vi "Request Data Persistence.vi"(6 "One Shot? (F)":bool, 7 "Initialize Persistence If None Found? (T)":bool=TRUE, 8 "error in (no error)":errorcluster, 9 "Data Type/Initial Value":variant, 10 "Datum Name":string, 11 "IObserver in":refnum<class "IObserver.lvclass">) -> (0 "error out":errorcluster, 2 "Subscription Policy":T1, 3 "IObserver out":refnum<class "IObserver.lvclass">)   [LabVIEW 2015, in "IObserver.lvlib" / "IObserver.lvclass"]
doc: "<License>\nCopyright © 2017 Composed Systems, LLC | All rights reserved\nwww.composed.io\n\nAuthor: Ethan Stern <ethan.stern@composed.io>\n\nThis software is provided \"AS IS\" WITHOUT WARRANTIES, either express or implied, AND IS FOR EDUCATIONAL PURPOSES ONLY.\n</License>"
uses:
  IObserver.lvclass
  IMediator/ISubscriptionPolicy/ISubscriptionPolicy Reference.ctl
  IMediator/ISubscriptionPolicy/ISubscriptionPolicy.lvclass
  <vilib>/ActorFramework/Actor/Actor.lvclass/Actor.ctl
  <vilib>/ActorFramework/Message Enqueuer/Message Enqueuer.lvclass/Message Enqueuer.ctl
  SubscriptionPolicy/ValueChangeSubscription/ValueChangeSubscription.lvclass/ValueChangeSubscription.ctl
  SubscriptionPolicy/OneShotSubscription/OneShotSubscription.lvclass/OneShotSubscription.ctl
  Transport/PersistToDiskTransport/PersistToDiskTransport.lvclass/PersistToDiskTransport.ctl
  IMediator/SubscriptionRequest/SubscriptionRequest.lvclass/SubscriptionRequest.ctl
  IObserver Messages/Subscribe Msg/Subscribe Msg.lvclass/Subscribe Msg.ctl
  <vilib>/ActorFramework/Message Enqueuer/Init from Existing Queue.vi
  <vilib>/ActorFramework/Message Enqueuer/Enqueue.vi
  <vilib>/Utility/error.llb/Clear Errors.vi
  <vilib>/ActorFramework/Message Priority Queue/Priority Enqueue.vi
  IObserver Messages/Subscribe Msg/Subscribe Msg.lvclass
  <vilib>/ActorFramework/Message Enqueuer/Message Enqueuer.lvclass
  IMediator/SubscriptionRequest/SubscriptionRequest.lvclass
  Transport/PersistToDiskTransport/PersistToDiskTransport.lvclass
  SubscriptionPolicy/OneShotSubscription/OneShotSubscription.lvclass
  SubscriptionPolicy/ValueChangeSubscription/ValueChangeSubscription.lvclass
  <vilib>/ActorFramework/Actor/Actor.lvclass
panel:
  in  "Persistence Folder Path":path
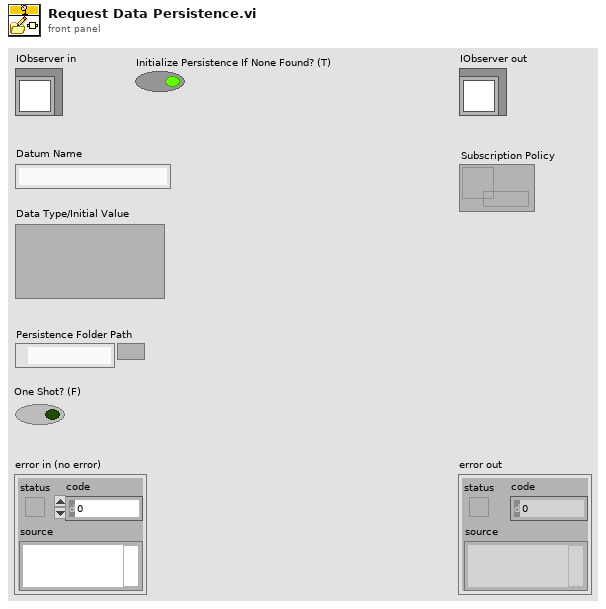
[diagram p1: front panel]
types:
  T1 = typedef "IMediator.lvlib/ISubscriptionPolicy.lvclass/ISubscriptionPolicy Reference.ctl" = refnum<data-value>
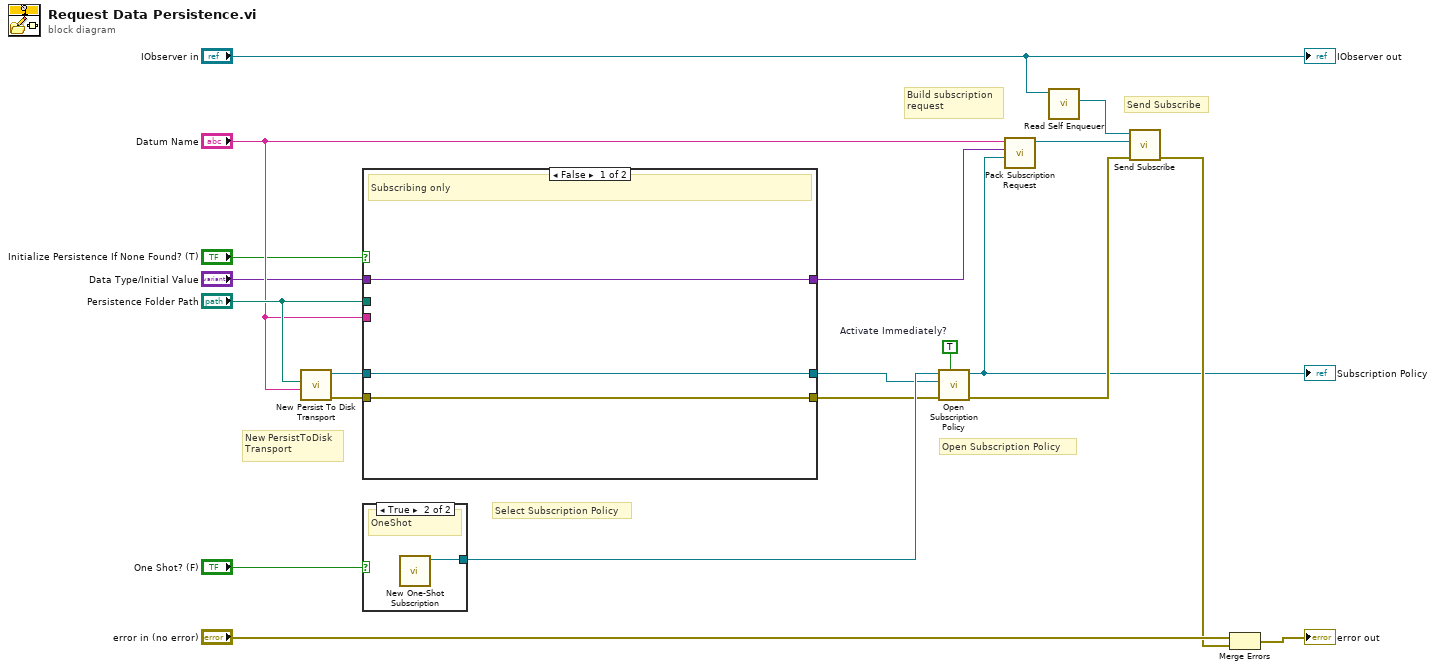
[diagram p0: block diagram]
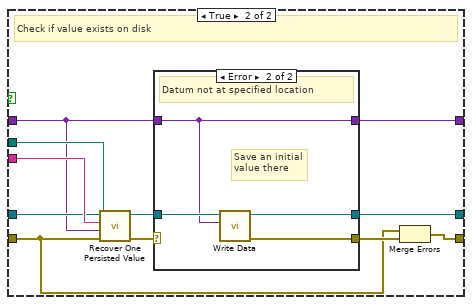
[diagram p2: hidden frame]
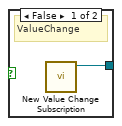
[diagram p4: hidden frame]
diagram:
  w12 = TRUE  # Activate Immediately?
  # "Open Subscription Policy"
  # "Select Subscription Policy"
  # "Send Subscribe"
  # "Build subscription\nrequest"
  # "New PersistToDisk\nTransport"
  n1 = call "New Persist To Disk Transport.vi"("Datum Name"="Datum Name", "Folder Path"="Persistence Folder Path") -> ("error out"=w6:errorcluster, "PersistToDiskTransport Out"=w2:refnum<class "PersistToDiskTransport.lvclass">)  [unwired: 8 in]
  n2 = case shown="False" "Initialize Persistence If None Found? (T)" {
    tunnel: "Persistence Folder Path" -> [_ w33]
    tunnel: "Datum Name" -> [_ w32]
    tunnel: "Data Type/Initial Value" -> [w23 w27]
    tunnel: w6 -> [w22 w24]
    tunnel: [w22 w25] -> w3
    tunnel: [w23 w26] -> w5
    tunnel: w2 -> [w21 w29]
    tunnel: [w21 w28] -> w1
    frame False {
      # "Subscribing only"
    }
    frame True {
      # "Check if value exists on disk"
      n3 = call "Recover One Persisted Value.vi"("error in (no error)"=w24, "Data Type"=w27, "Datum Name"=w32, "Folder Path"=w33) -> ("error out"=w31:errorcluster)  [unwired: 6 in, 1 out]
      n4 = case shown="Error" w31 {
        selector: w31 -> [w34 _]
        tunnel: [w34 w40] -> w30
        tunnel: w29 -> [w35 w39]
        tunnel: [w35 w38] -> w28
        tunnel: w27 -> [w36 w37]
        tunnel: [w36 w37] -> w26
        frame No Error {
          # "Do nothing more"
          # "Datum already on disk"
        }
        frame Error {
          # "Save an initial\nvalue there"
          # "Datum not at specified location"
          n5 = call-dynamic "Write Data.vi"("Value"=w37, "PersistToDiskTransport In"=w39) -> ("error out"=w40:errorcluster, "PersistToDiskTransport Out"=w38:refnum<class "PersistToDiskTransport.lvclass">)  [unwired: 8 in]
        }
      }
      n6 = Merge Errors(w24, w30) -> (w25:errorcluster)
    }
  }
  n7 = case shown="True" "One Shot? (F)" {
    tunnel: [w41 w42] -> w10
    frame False {
      # "ValueChange"
      n8 = call "New Value Change Subscription.vi"() -> ("ValueChangeSubscription Out"=w41:refnum<class "ValueChangeSubscription.lvclass">)  [unwired: 11 in]
    }
    frame True {
      # "OneShot"
      n9 = call "New One-Shot Subscription.vi"() -> ("OneShotSubscription Out"=w42:refnum<class "OneShotSubscription.lvclass">)  [unwired: 11 in]
    }
  }
  n10 = call "Open Subscription Policy.vi"("Activate? (T)"=w12, "error in (no error)"=w3, "Transport"=w1, "SubscriptionPolicy"=w10) -> ("error out"=w15:errorcluster, "Subscription Policy"=w11:T1)  [unwired: 6 in]
  "Subscription Policy" <- w11
  n11 = call "Pack Subscription Request.vi"("Subscription Policy"=w11, "Type"=w5, "Datum Name"="Datum Name") -> ("SubscriptionRequest"=w16:refnum<class "SubscriptionRequest.lvclass">)  [unwired: 8 in]
  n12 = call <vilib>:"Read Self Enqueuer.vi"("Actor"="IObserver in") -> ("Self Enqueuer"=w13:refnum<class "Message Enqueuer.lvclass">)  [unwired: 10 in]
  n13 = call "Send Subscribe.vi"("error in (no error)"=w15, "SubscriptionRequest"=w16, "Message Enqueuer"=w13) -> ("error out"=w14:errorcluster)  [unwired: 7 in, 1 out]
  n14 = Merge Errors("error in (no error)", w14) -> (→"error out":errorcluster)
  "IObserver out" <- "IObserver in"
